vi "array2cluster.vi"() -> ()   [LabVIEW 2021]
panel:
  out "Cluster output":cluster{"X":dbl, "Y":dbl, "Index":dbl}
  in  "Index select":u16
  in  "Y Coordinates":dbl[](array[numeric])
  in  "X coordinates":dbl[](array[numeric])
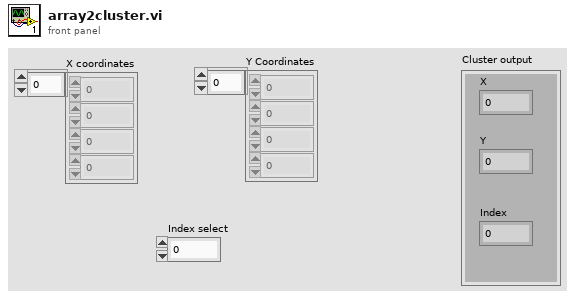
[diagram p1: front panel]
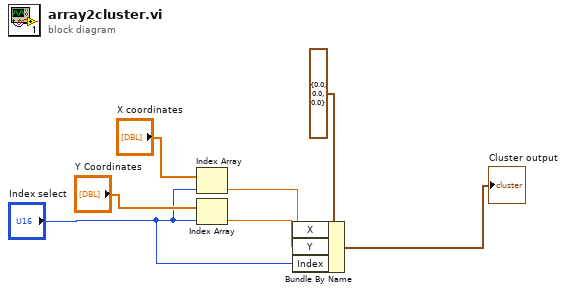
[diagram p0: block diagram]
diagram:
  n1 = Index Array(array="X coordinates", index="Index select") -> (element=w3:dbl)
  n2 = Index Array(array="Y Coordinates", index="Index select") -> (element=w4:dbl)
  n3 = Bundle By Name(cluster=cluster{"X":dbl, "Y":dbl, "Index":dbl} {"X"=0.0, "Y"=0.0, "Index"=0.0} ("Cluster output"), "X"=w3, "Y"=w4, "Index"="Index select") -> (→"Cluster output":cluster{"X":dbl, "Y":dbl, "Index":dbl})
